vi "Z900_navX_Internal_UpdateDevice.vi"(8 "error in (no error)":errorcluster, 10 "Interface TypeDefs":T1 {"I2CDevRef"."Device Address" format="%.0x"}, 11 "navX Device":T7={"Interface"={"Protocol"=enum."SERIAL", "Update Rate (4Hz-100Hz)"=4, "navX Open TypeDef"=variant}, "Notify Packet"=refnum, "Loop VI Refnum"=refnum, "Ready to Close Occurrence Refnum"=refnum} {"Interface"."Update Rate (4Hz-100Hz)" min=4 max=60 step=1}) -> (0 "error out":errorcluster, 2 "Interface TypeDefs":T1 {"I2CDevRef"."Device Address" format="%.0x"}, 3 "navX Device":T7={"Interface"={"Protocol"=enum."SERIAL", "Update Rate (4Hz-100Hz)"=4, "navX Open TypeDef"=variant}, "Notify Packet"=refnum, "Loop VI Refnum"=refnum, "Ready to Close Occurrence Refnum"=refnum} {"Interface"."Update Rate (4Hz-100Hz)" min=4 max=60 step=1})   [LabVIEW 2015, in "navX Library v2.lvlib"]
doc: "This navX VI handles updating rate and serial protocol for the navX.\nTHIS VI SHOULD NOT BE CALLED BY THE USER!"
uses:
  navX Library v2.lvlib
  _TypeDefs/Z900_navX_DeviceTypeDef.ctl
  _TypeDefs/Z900_navX_ProtocolTypeDef.ctl
  _TypeDefs/Z900_navX_NotifyPacketTypeDef.ctl
  _TypeDefs/Z900_navX_ActionTypeDef.ctl
  _TypeDefs/Z900_navX_InterfaceTypeDef.ctl
  <vilib>/Rock Robotics/WPI/SerialPort/WPI_SerialPortRef.ctl
  <vilib>/Rock Robotics/WPI/I2C/WPI_I2CDevRef.ctl
  <vilib>/Rock Robotics/SystemInterfaces/i2clib/i2c_bus.ctl
  <vilib>/Rock Robotics/WPI/SPI/WPI_SPIDevRef.ctl
  <vilib>/Rock Robotics/SystemInterfaces/spilib/spi_bus.ctl
  _TypeDefs/navX Open TypeDefs/Z900_navX_OpenTypeDef_Serial.ctl
  _NI WPI Serial USB/WPI_SerialPort_USB.ctl
  _TypeDefs/Z900_navX_SerialStreamTypeDef.ctl
  _TypeDefs/navX Open TypeDefs/Z900_navX_OpenTypeDef_I2C.ctl
  _TypeDefs/Z900_navX_DeviceRegisters.ctl
  _TypeDefs/navX Open TypeDefs/Z900_navX_OpenTypeDef_SPI.ctl
  _NI WPI Serial USB/_NI WPI Serial USB.lvlib
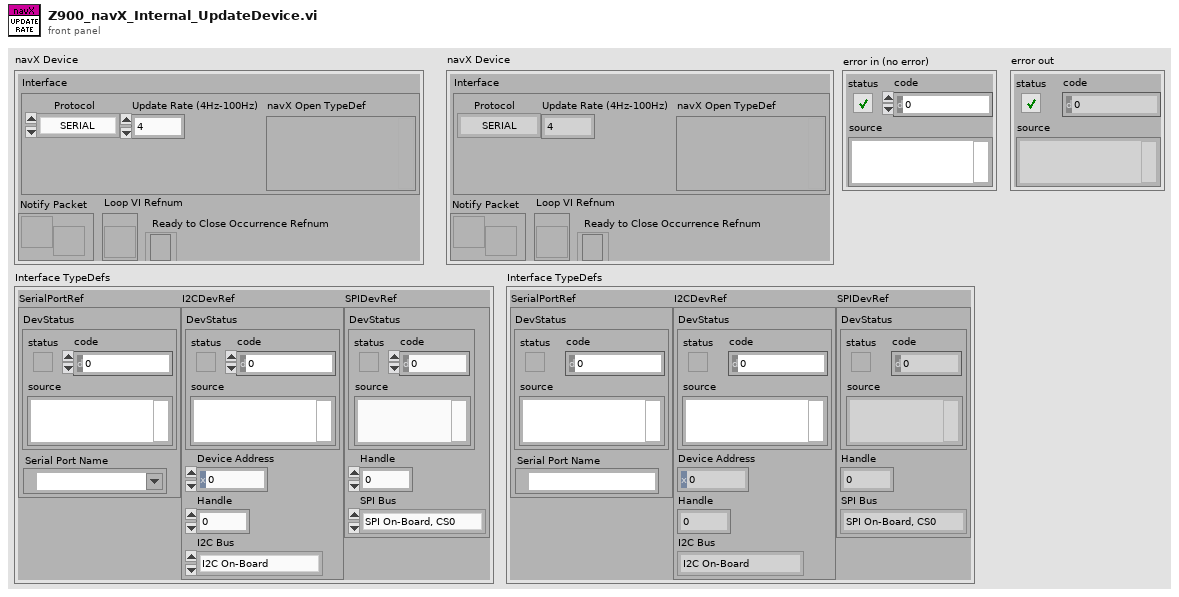
[diagram p1: front panel]
types:
  T1 = typedef "navX Library v2.lvlib/Z900_navX_InterfaceTypeDef.ctl" = cluster{"SerialPortRef":T2, "I2CDevRef":T3, "SPIDevRef":T5}
  T2 = typedef "WPI_SerialPortRef.ctl" = cluster{"DevStatus":errorcluster, "Serial Port Name":refnum<visa-resource-name>}
  T3 = typedef "WPI_I2CDevRef.ctl" = cluster{"DevStatus":errorcluster, "Device Address":u8, "Handle":i32, "I2C Bus":T4}
  T4 = typedef "i2c_bus.ctl" = enum16{"I2C On-Board", "I2C MXP", "Invalid"}
  T5 = typedef "WPI_SPIDevRef.ctl" = cluster{"DevStatus":errorcluster, "Handle":i32, "SPI Bus":T6}
  T6 = typedef "spi_bus.ctl" = enum16{"SPI On-Board, CS0", "SPI On-Board, CS1", "SPI On-Board, CS2", "SPI On-Board, CS3", "SPI MXP", "Invalid"}
  T7 = typedef "navX Library v2.lvlib/Z900_navX_DeviceTypeDef.ctl" = cluster{"Interface":cluster{"Protocol":T8, "Update Rate (4Hz-100Hz)":u8, "navX Open TypeDef":variant}, "Notify Packet":refnum<notifier>, "Loop VI Refnum":refnum<vi>, "Ready to Close Occurrence Refnum":refnum<k4>}
  T8 = typedef "navX Library v2.lvlib/Z900_navX_ProtocolTypeDef.ctl" = enum16{"SERIAL", "I2C", "SPI"}
  T9 = typedef "navX Library v2.lvlib/Z900_navX_OpenTypeDef_Serial.ctl" = cluster{"Serial Port":T10, "Stream Type":T11}
  T10 = typedef "_NI WPI Serial USB.lvlib/WPI_SerialPort_USB.ctl" = enum16{"Onboard RS-232", "MXP TTL", "USB"}
  T11 = typedef "navX Library v2.lvlib/Z900_navX_SerialStreamTypeDef.ctl" = enum16{"YRPH", "Quaterinons", "Gyro/Raw", "AHRS", "AHRSAndPositioning"}
  T12 = typedef "navX Library v2.lvlib/Z900_navX_OpenTypeDef_I2C.ctl" = cluster{"I2C Bus":T4}
  T13 = typedef "navX Library v2.lvlib/Z900_navX_OpenTypeDef_SPI.ctl" = cluster{"SPI Bus":T6, "Clock Rate (Hz)":dbl}
  T14 = typedef "navX Library v2.lvlib/Z900_navX_DeviceRegisters.ctl" = u8
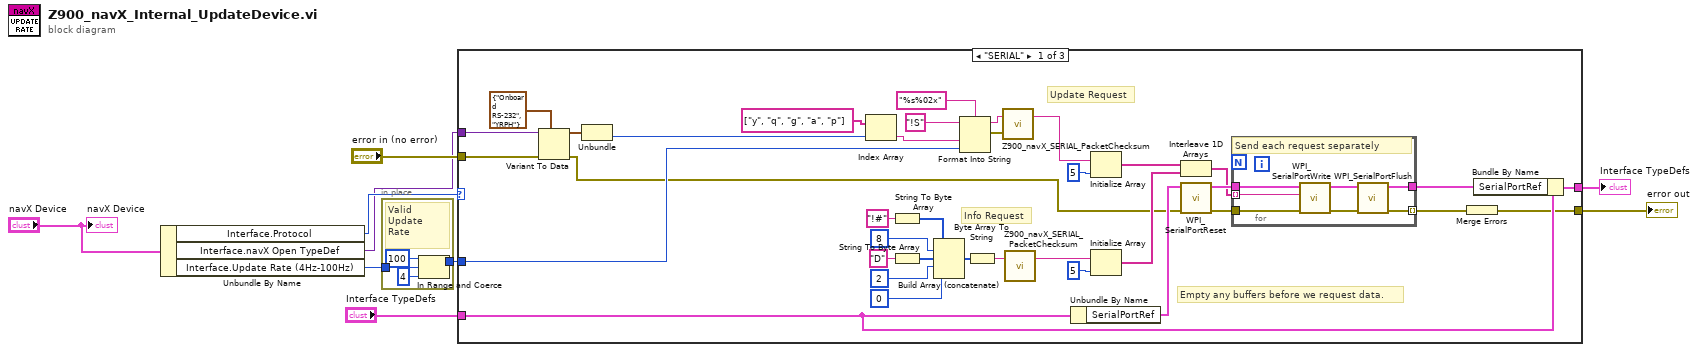
[diagram p0: block diagram]
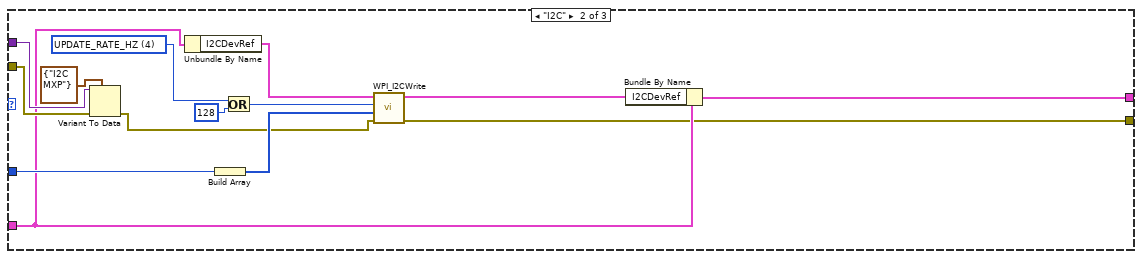
[diagram p2: hidden frame]
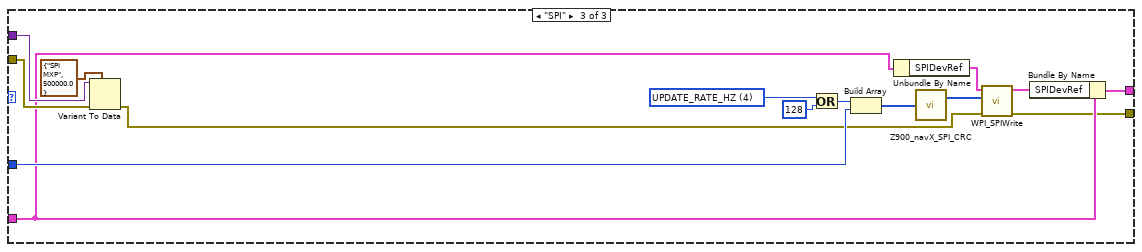
[diagram p3: hidden frame]
diagram:
  n1 = Unbundle By Name("navX Device") -> ("Interface.Protocol"=w8:T8, "Interface.navX Open TypeDef"=w4:variant, "Interface.Update Rate (4Hz-100Hz)"=w3:u8)
  n2 = in-place {
    in-place-border: w3 -> [w13]
    in-place-border: [w10] -> w2
    # "Valid\nUpdate\nRate"
    n3 = In Range and Coerce(upper limit=u8 100, x=w13, lower limit=u8 4) -> (coerced(x)=w10:u8)  [unwired: 1 out]
  }
  n4 = case shown="\"SERIAL\"" w8 {
    tunnel: w4 -> [w50 w71 w86]
    tunnel: "error in (no error)" -> [w48 w69 w84]
    tunnel: "Interface TypeDefs" -> [w45 w62 w76]
    tunnel: w2 -> [w43 w65 w78]
    tunnel: [w44 w60 w74] -> w5
    tunnel: [w30 w58 w72] -> w1
    frame "SERIAL" {
      # "Info Request"
      # "Update Request"
      # "Empty any buffers before we request data."
      n5 = Variant To Data(error in=w48, type=T9 {"Serial Port"=enum."Onboard RS-232", "Stream Type"=enum."YRPH"} ("navX Serial Open"), Variant=w50) -> (data=w47:T9, error out=w29:errorcluster)
      n6 = Unbundle(w47) -> ("Stream Type"=w46:T11)  [unwired: 1 out]
      n7 = Index Array(array=string[] ["y", "q", "g", "a", "p"], index=w46) -> (element=w23:string)
      n8 = String To Byte Array(string="!#" ("initial string")) -> (unsigned byte array=w20:u8[])
      n9 = String To Byte Array(string="D" ("initial string")) -> (unsigned byte array=w18:u8[])
      n10 = Build Array (concatenate)(w20, 8, w18, 2, 0) -> (w15:i32[])
      n11 = Format Into String(format string="%s%02x", initial string="!S", w23, w43) -> (resulting string=w26:string, error out=w27:errorcluster)  [unwired: 1 in]
      n12 = Byte Array To String(unsigned byte array=w15) -> (string=w14:string)
      n13 = call "Z900_navX_SERIAL_PacketChecksum.vi"("error in (no error)"=w27, "Packet"=w26) -> ("Terminated Packet"=w38:string)  [unwired: 1 out]
      n14 = call "Z900_navX_SERIAL_PacketChecksum.vi"("Packet"=w14) -> ("Terminated Packet"=w36:string)  [unwired: 1 in, 1 out]
      n15 = Unbundle By Name(w45) -> ("SerialPortRef"=w41:T2)
      n16 = Initialize Array(w38, 5 ("dimension size")) -> (w35:string[])
      n17 = Initialize Array(w36, 5 ("dimension size")) -> (w34:string[])
      n18 = Interleave 1D Arrays(w35, w34) -> (w33:string[])
      n19 = call <vilib>:"WPI_SerialPortReset.vi"("error in (no error)"=w29, "SerialPortRef"=w41) -> ("error out"=w39:errorcluster, "SerialPortRef"=w40:T2)  [unwired: 8 in]
      n20 = for {
        tunnel: w39 -> [w54]
        tunnel: w33 -> [w53] mode=indexing
        tunnel: [w51] -> w31 mode=indexing
        tunnel: w40 -> [w55]
        tunnel: [w52] -> w32
        # "Send each request separately"
        n21 = call <vilib>:"WPI_SerialPortWrite.vi"("error in (no error)"=w54, "Buffer"=w53, "SerialPortRef"=w55) -> ("error out"=w56:errorcluster, "SerialPortRef"=w57:T2)  [unwired: 6 in, 1 out]
        n22 = call <vilib>:"WPI_SerialPortFlush.vi"("error in (no error)"=w56, "SerialPortRef"=w57) -> ("error out"=w51:errorcluster, "SerialPortRef"=w52:T2)  [unwired: 8 in]
      }
      n23 = Merge Errors(w31) -> (w30:errorcluster)
      n24 = Bundle By Name(cluster=w45, "SerialPortRef"=w32) -> (w44:T1)
    }
    frame "I2C" {
      w66 = T14 4 items=["WHOAMI"=0, "HW_REV"=1, "FW_VER_MAJOR"=2, "FW_VER_MINOR"=3, "UPDATE_RATE_HZ"=4, "ACCEL_FSR_G"=5, "GYRO_FSR_DPS"=6, "OP_STATUS"=8, "CAL_STATUS"=9, "SELFTEST_STATUS"=10, "CAPABILITY_FLAGS_L"=11, "CAPABILITY_FLAGS_H"=12, "SENSOR_STATUS"=16, "TIMESTAMP"=18, "YAW"=22, "ROLL"=24, "PITCH"=26, "HEADING"=28, "FUSED_HEADING"=30, "ALTITUDE_I"=32, "ALTITUDE_D"=34, "LINERA_ACC_X"=36, "LINERA_ACC_Y"=38, "LINERA_ACC_Z"=40, "QUAT_W"=42, "QUAT_X"=44, "QUAT_Y"=46, "QUAT_Z"=48, "MPU_TEMP_C"=50, "GYRO_X"=52, "GYRO_Y"=54, "GYRO_Z"=56, "ACC_X"=58, "ACC_Y"=60, "ACC_Z"=62, "MAG_X"=64, "MAG_Y"=66, "MAG_Z"=68, "PRESSURE_I"=70, "PRESSURE_D"=72, "PRESSURE_TEMP"=74, "YAW_OFFSET"=76, "QUAT_OFFSET_W"=78, "QUAT_OFFSET_X"=80, "QUAT_OFFSET_Y"=82, "QUAT_OFFSET_Z"=84, "INTEGRATION_CONTROL"=86, "VELOCITY_X"=88, "VELOCITY_Y"=92, "VELOCITY_Z"=96, "DISPLACMENT_X"=100, "DISPLACMENT_Y"=104, "DISPLACEMENT_Z"=108] ("Device Register")
      n25 = Variant To Data(error in=w69, type=T12 {"I2C Bus"=enum."I2C MXP"} ("navX I2C Open"), Variant=w71) -> (error out=w59:errorcluster)  [unwired: 1 out]
      n26 = Unbundle By Name(w62) -> ("I2CDevRef"=w63:T3)
      n27 = Build Array(w65) -> (w64:u8[])
      n28 = Or(x=w66, y=u8 128) -> (x .or. y?=w68:T14)
      n29 = call <vilib>:"WPI_I2CWrite.vi"("error in (no error)"=w59, "I2CDataToSend"=w64, "I2CRegister"=w68, "I2CDevRef"=w63) -> ("error out"=w58:errorcluster, "I2CDevRef"=w61:T3)  [unwired: 6 in]
      n30 = Bundle By Name(cluster=w62, "I2CDevRef"=w61) -> (w60:T1)
    }
    frame "SPI" {
      w80 = T14 4 items=["WHOAMI"=0, "HW_REV"=1, "FW_VER_MAJOR"=2, "FW_VER_MINOR"=3, "UPDATE_RATE_HZ"=4, "ACCEL_FSR_G"=5, "GYRO_FSR_DPS"=6, "OP_STATUS"=8, "CAL_STATUS"=9, "SELFTEST_STATUS"=10, "CAPABILITY_FLAGS_L"=11, "CAPABILITY_FLAGS_H"=12, "SENSOR_STATUS"=16, "TIMESTAMP"=18, "YAW"=22, "ROLL"=24, "PITCH"=26, "HEADING"=28, "FUSED_HEADING"=30, "ALTITUDE_I"=32, "ALTITUDE_D"=34, "LINERA_ACC_X"=36, "LINERA_ACC_Y"=38, "LINERA_ACC_Z"=40, "QUAT_W"=42, "QUAT_X"=44, "QUAT_Y"=46, "QUAT_Z"=48, "MPU_TEMP_C"=50, "GYRO_X"=52, "GYRO_Y"=54, "GYRO_Z"=56, "ACC_X"=58, "ACC_Y"=60, "ACC_Z"=62, "MAG_X"=64, "MAG_Y"=66, "MAG_Z"=68, "PRESSURE_I"=70, "PRESSURE_D"=72, "PRESSURE_TEMP"=74, "YAW_OFFSET"=76, "QUAT_OFFSET_W"=78, "QUAT_OFFSET_X"=80, "QUAT_OFFSET_Y"=82, "QUAT_OFFSET_Z"=84, "INTEGRATION_CONTROL"=86, "VELOCITY_X"=88, "VELOCITY_Y"=92, "VELOCITY_Z"=96, "DISPLACMENT_X"=100, "DISPLACMENT_Y"=104, "DISPLACEMENT_Z"=108] ("Device Register")
      n31 = Variant To Data(error in=w84, type=T13 {"SPI Bus"=enum."SPI MXP", "Clock Rate (Hz)"=500000.0} ("navX SPI Open"), Variant=w86) -> (error out=w73:errorcluster)  [unwired: 1 out]
      n32 = Or(x=w80, y=u8 128) -> (x .or. y?=w81:T14)
      n33 = Build Array(w81, w78) -> (w82:T14[])
      n34 = Unbundle By Name(w76) -> ("SPIDevRef"=w77:T5)
      n35 = call "Z900_navX_SPI_CRC.vi"("Message"=w82) -> ("Message with CRC"=w83:u8[])  [unwired: 1 out]
      n36 = call <vilib>:"WPI_SPIWrite.vi"("error in (no error)"=w73, "Data To Send"=w83, "SPIDevRef"=w77) -> ("error out"=w72:errorcluster, "SPIDevRef"=w75:T5)  [unwired: 6 in, 1 out]
      n37 = Bundle By Name(cluster=w76, "SPIDevRef"=w75) -> (w74:T1)
    }
  }
  "error out" <- w1
  "Interface TypeDefs" <- w5
  "navX Device" <- "navX Device"
